vi "Q-Preview.vi"(7 "Queue Type":T1, 8 "error in":errorcluster, 9 "timeout in ms (-1)":i32=-1, 11 "Q Name":string) -> (0 "error out":errorcluster, 1 "Index":i32, 2 "Analog Data":waveform(dbl)[](array[waveform]), 3 "Digital Data":digitalwaveform[](array[waveform]), 4 "timed out?":bool, 5 "Variant Data":variant[](array[variant]))   [LabVIEW 2016]
uses:
  PSDAQEG_Task Queue Type.ctl
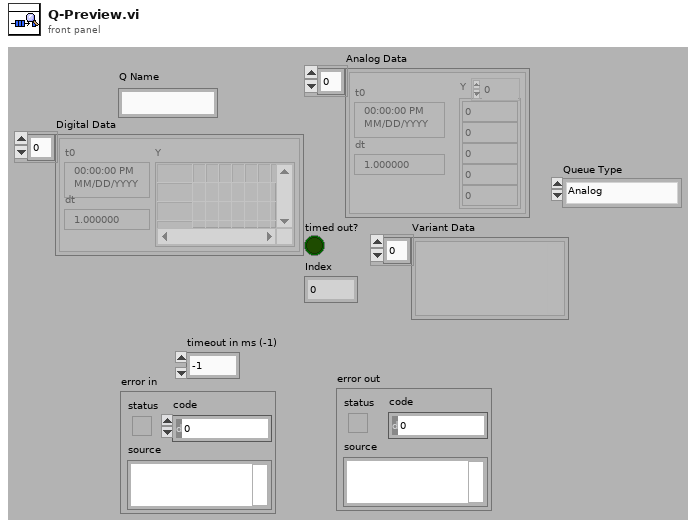
[diagram p1: front panel]
types:
  T1 = typedef "PSDAQEG_Task Queue Type.ctl" = enum16{"Analog", "Digital", "Variant"}
  T2 = cluster{"max queue size (-1, unlimited)":i32, "Waveform":waveform(dbl)[]}
  T3 = cluster{"max queue size (-1, unlimited)":i32, digitalwaveform[]}
  T4 = cluster{"max queue size (-1, unlimited)":i32, variant[]}
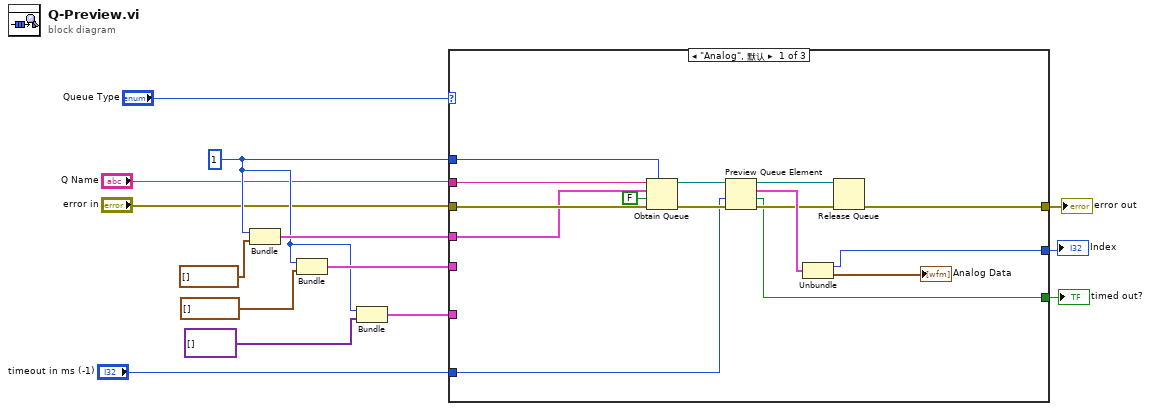
[diagram p0: block diagram]
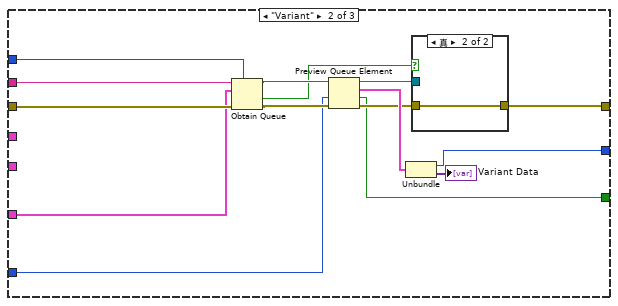
[diagram p2: hidden frame]
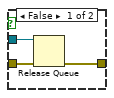
[diagram p3: hidden frame]
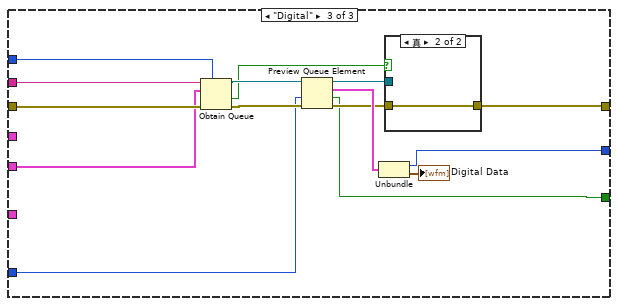
[diagram p4: hidden frame]
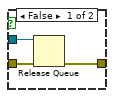
[diagram p5: hidden frame]
diagram:
  w8 = 1 ("max queue size (-1, unlimited)")
  n1 = Bundle("max queue size (-1, unlimited)"=w8, "Waveform"=waveform(dbl)[] []) -> (w10:T2)  [unwired: 1 in]
  n2 = Bundle("max queue size (-1, unlimited)"=w8, digitalwaveform[] []) -> (w11:T3)  [unwired: 1 in]
  n3 = Bundle("max queue size (-1, unlimited)"=w8, variant[] []) -> (w7:T4)  [unwired: 1 in]
  n4 = case shown="\"Analog\", 默认" "Queue Type" {
    tunnel: "Q Name" -> [w28 w43 w63]
    tunnel: "error in" -> [w29 w44 w62]
    tunnel: w8 -> [w27 w42 w61]
    tunnel: w11 -> [_ _ w60]
    tunnel: [w18 w31 w51] -> w3
    tunnel: w10 -> [w26 _ _]
    tunnel: w7 -> [_ w41 _]
    tunnel: "timeout in ms (-1)" -> [w16 w35 w54]
    tunnel: [w19 w32 w52] -> w2
    tunnel: [w17 w33 w53] -> w1
    frame "Analog", Default {
      n5 = Obtain Queue(max queue size (-1, unlimited)=w27, name (unnamed)=w28, element data type=w26, create if not found? (T)=FALSE, error in (no error)=w29) -> (queue out=w22:refnum<queue>, error out=w21:errorcluster)  [unwired: 1 out]
      n6 = Preview Queue Element(queue=w22, timeout in ms (-1)=w16, error in (no error)=w21) -> (queue out=w23:refnum<queue>, element=w25:T2, timed out?=w17:bool, error out=w24:errorcluster)
      n7 = Unbundle(w25) -> ("max queue size (-1, unlimited)"=w19:i32, "Waveform"=→"Analog Data":waveform(dbl)[])
      n8 = Release Queue(queue=w23, error in (no error)=w24) -> (error out=w18:errorcluster)  [unwired: 1 in, 2 out]
    }
    frame "Variant" {
      n9 = Obtain Queue(max queue size (-1, unlimited)=w42, name (unnamed)=w43, element data type=w41, error in (no error)=w44) -> (queue out=w36:refnum<queue>, created new?=w34:bool, error out=w37:errorcluster)  [unwired: 1 in]
      n10 = Preview Queue Element(queue=w36, timeout in ms (-1)=w35, error in (no error)=w37) -> (queue out=w38:refnum<queue>, element=w40:T4, timed out?=w33:bool, error out=w39:errorcluster)
      n11 = Unbundle(w40) -> ("max queue size (-1, unlimited)"=w32:i32, →"Variant Data":variant[])
      n12 = case shown="真" w34 {
        tunnel: w38 -> [w47 _]
        tunnel: w39 -> [w46 w48]
        tunnel: [w45 w48] -> w31
        frame False {
          n13 = Release Queue(queue=w47, error in (no error)=w46) -> (error out=w45:errorcluster)  [unwired: 1 in, 2 out]
        }
        frame True {
        }
      }
    }
    frame "Digital" {
      n14 = Obtain Queue(max queue size (-1, unlimited)=w61, name (unnamed)=w63, element data type=w60, error in (no error)=w62) -> (queue out=w56:refnum<queue>, created new?=w50:bool, error out=w55:errorcluster)  [unwired: 1 in]
      n15 = Preview Queue Element(queue=w56, timeout in ms (-1)=w54, error in (no error)=w55) -> (queue out=w57:refnum<queue>, element=w59:T3, timed out?=w53:bool, error out=w58:errorcluster)
      n16 = Unbundle(w59) -> ("max queue size (-1, unlimited)"=w52:i32, →"Digital Data":digitalwaveform[])
      n17 = case shown="真" w50 {
        tunnel: w57 -> [w66 _]
        tunnel: w58 -> [w65 w67]
        tunnel: [w64 w67] -> w51
        frame False {
          n18 = Release Queue(queue=w66, error in (no error)=w65) -> (error out=w64:errorcluster)  [unwired: 1 in, 2 out]
        }
        frame True {
        }
      }
    }
  }
  "error out" <- w3
  "timed out?" <- w1
  "Index" <- w2
